vi "Configure Timer (Absolute).vi"(0 "VISA resource name":refnum<visa-resource-name>, 1 "Hour (0)":i32 min=0 max=23, 2 "Minute (0)":i32 min=0 max=59, 5 "Timer No. (1)":i32=1 min=1 max=12, 7 "Interval (1h)":u16(ring)=11 items=["1min", "2min", "3min", "4min", "5min", "6min", "10min", "12min", "15min", "20min", "30min", "1h", "2h", "3h", "4h", "6h", "8h", "12h", "24h"], 11 "error in (no error)":errorcluster) -> (4 "VISA resource name out":refnum<visa-resource-name>, 6 "Timer No.":i32, 15 "error out":errorcluster)   [LabVIEW 2020, in "Yokogawa GX Series.lvlib"]
doc: "Sets the absolute timer.\n\nCommand: STimer"
uses:
  <instrlib>/Yokogawa GX Series/Yokogawa GX Series.lvlib
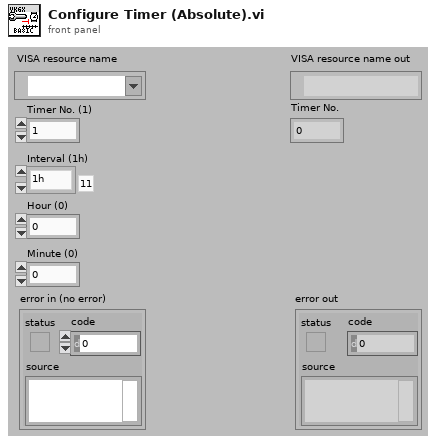
[diagram p1: front panel]
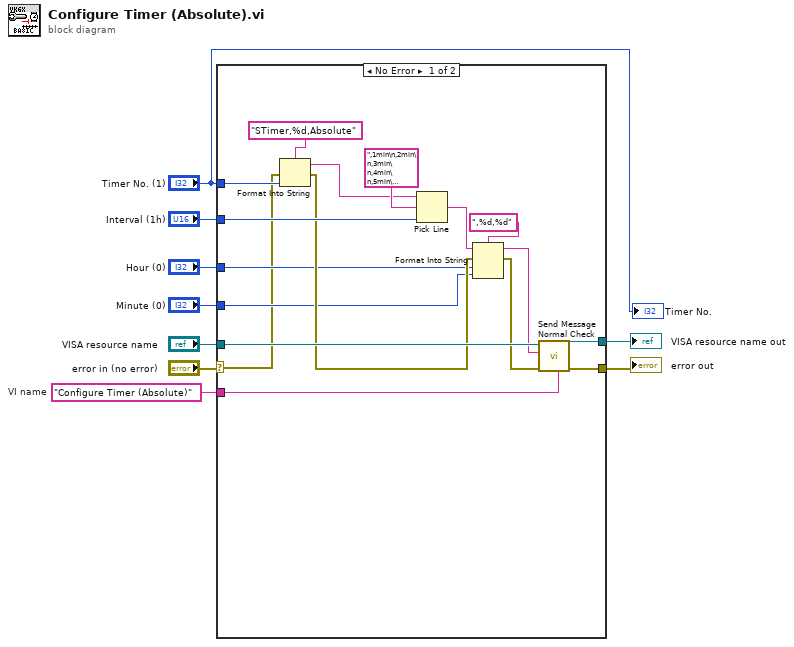
[diagram p0: block diagram]
diagram:
  w9 = "Configure Timer (Absolute)"  # VI name
  n1 = case shown="No Error" "error in (no error)" {
    selector: "error in (no error)" -> [w10 w27]
    tunnel: w9 -> [w26 _]
    tunnel: [w25 w28] -> w8
    tunnel: [w24 w27] -> w7
    tunnel: "VISA resource name" -> [w22 w28]
    tunnel: "Timer No. (1)" -> [w21 _]
    tunnel: "Interval (1h)" -> [w18 _]
    tunnel: "Hour (0)" -> [w12 _]
    tunnel: "Minute (0)" -> [w11 _]
    frame No Error {
      n2 = Format Into String(format string="STimer,%d,Absolute", error in=w10, w21) -> (resulting string=w19:string, error out=w14:errorcluster)  [unwired: 1 in]
      n3 = Pick Line(string ("")=w19, multi-line string=",1min\n,2min\n,3min\n,4min\n,5min\n,6min\n,10min\n,12min\n,15min\n,20min\n,30min\n,1h\n,2h\n,3h\n,4h\n,6h\n,8h\n,12h\n,24h", line index=w18) -> (output string=w17:string)
      n4 = Format Into String(format string=",%d,%d", initial string=w17, error in=w14, w12, w11) -> (resulting string=w15:string, error out=w13:errorcluster)
      n5 = call <instrlib>:"Send Message Normal Check.vi"("Source (\"\")"=w26, "error in (no error)"=w13, "Send Message (\"\")"=w15, "VISA resource name"=w22) -> ("error out"=w24:errorcluster, "VISA resource name out"=w25:refnum<visa-resource-name>)  [unwired: 2 in, 4 out]
    }
    frame Error {
    }
  }
  "error out" <- w7
  "VISA resource name out" <- w8
  "Timer No." <- "Timer No. (1)"
